vi "Set Turbo Valve Settings.vi"(10 "Turbo Valve Settings":T1={"ROT Bias"=70, "Minimum Voltage"=0.0, "Maximum Voltage"=4.096, "Off Value"=0.0} {"Off Value" format="%.3f"; "Maximum Voltage" format="%.3f"; "Minimum Voltage" format="%.3f"; "ROT Bias" max=127 step=1}, 11 "ILC Actuator Cylinder in":refnum<class "ILC Actuator Cylinder.lvclass">) -> (3 "ILC Actuator Cylinder out":refnum<class "ILC Actuator Cylinder.lvclass">)   [LabVIEW 2015, in "ILC Actuator Cylinder.lvclass"]
uses:
  ILC Actuator Cylinder.lvclass
  Typedefs/Turbo Valve Settings.ctl
  ILC Actuator Cylinder.lvclass/ILC Actuator Cylinder.ctl
  Typedefs/FAMT Typedefs.lvlib
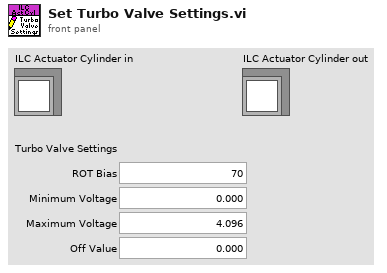
[diagram p1: front panel]
types:
  T1 = typedef "FAMT Typedefs.lvlib/Turbo Valve Settings.ctl" = cluster{"ROT Bias":u8, "Minimum Voltage":dbl, "Maximum Voltage":dbl, "Off Value":dbl}
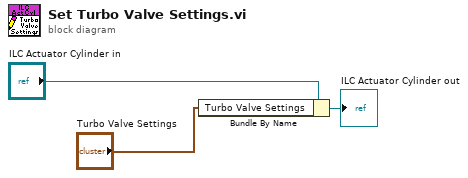
[diagram p0: block diagram]
diagram:
  n1 = Bundle By Name(cluster="ILC Actuator Cylinder in", "Turbo Valve Settings"="Turbo Valve Settings") -> (→"ILC Actuator Cylinder out":refnum<class "ILC Actuator Cylinder.lvclass">)
